vi "Split String Tree.vi"(1 "Ignore Pattern":string, 4 "Split Pattern":string, 6 "Input String":string) -> (2 "Split String":string[](array[string]))   [LabVIEW 2020, in "NI_VIAnCFGDataStructure.lvlib" / "Tree.lvclass"]
doc: "Splits a string at a pattern into an array of strings.\n\n<B>Input String</B> - The string to split.\n<B>Split Pattern</B> - The regular expression to split the string at.\n<B>Ignore Pattern</B> - Defines when a split pattern should be ignored.\n<B>Split String</B> - The array of elements between found instances of <B>Split Pattern</B> in <B>Input String</B>."
uses:
  <vilib>/addons/analyzer/VIAnCFGDataStructure/Tree Manager/Tree.lvclass
  <vilib>/regexp/Match Regular Expression.xnode
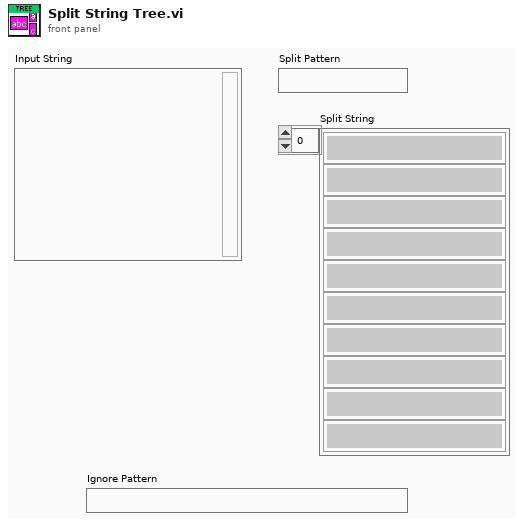
[diagram p1: front panel]
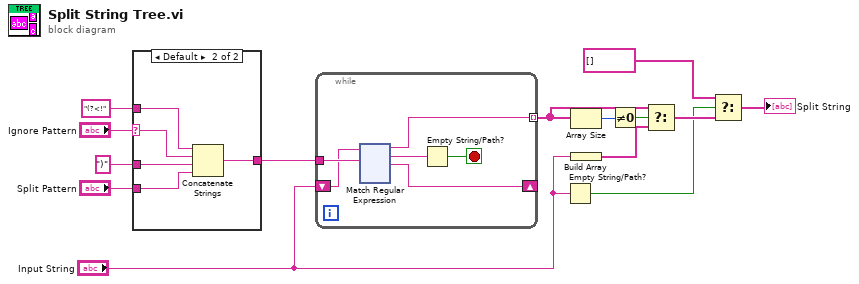
[diagram p0: block diagram]
diagram:
  n1 = case shown="Default" "Ignore Pattern" {
    selector: "Ignore Pattern" -> [_ w16]
    tunnel: "(?<!" ("string") -> [_ w20]
    tunnel: [w15 w19] -> w4
    tunnel: ")" ("string") -> [_ w18]
    tunnel: "Split Pattern" -> [w15 w17]
    frame "" {
    }
    frame Default {
      n2 = Concatenate Strings(w20, w16, w18, w17) -> (w19:string)
    }
  }
  n3 = while {
    tunnel: [w25] -> w11 mode=indexing
    shift-right: [w23] -> _
    shift-left: "Input String" -> [w21]
    tunnel: w4 -> [w22]
    stop <- w26 stop-if-true
    n4 = xnode "Match Regular Expression"("input string"=w21, "regular expression"=w22) -> ("before match"=w25:string, "whole match"=w24:string, "after match"=w23:string)  [unwired: 4 in, 2 out]
    n5 = Empty String/Path?(string/path=w24) -> (empty?=w26:bool)
  }
  n6 = Empty String/Path?(string/path="Input String") -> (empty?=w8:bool)
  n7 = Array Size(array=w11) -> (size(s)=w14:i32)
  n8 = Build Array("Input String") -> (w12:string[])
  n9 = Not Equal To 0?(x=w14) -> (x != 0?=w13:bool)
  n10 = Select(t=w11, s=w13, f=w12) -> (s? t:f=w9:string[])
  n11 = Select(t=string[] [], s=w8, f=w9) -> (s? t:f=→"Split String":string[])
